vi "Read Component.vi"(6 "Create if non-existent? (F)":bool, 8 "error in (no error)":errorcluster, 10 "Qualified Path":string, 11 "Attribute.Identity in":refnum<class "Attribute.Identity.lvclass">) -> (0 "error out":errorcluster, 2 "Component":string, 3 "Attribute.Identity out":refnum<class "Attribute.Identity.lvclass">)   [LabVIEW 2013, in "Attribute.Identity.lvclass"]
uses:
  Attribute.Identity.lvclass
  Attribute.Identity.lvclass/Attribute.Identity.ctl
  <vilib>/Utility/MD5Checksum.llb/MD5Checksum string.vi
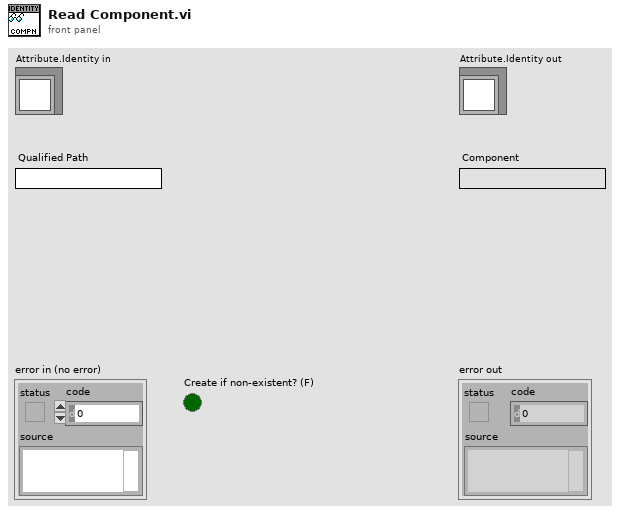
[diagram p1: front panel]
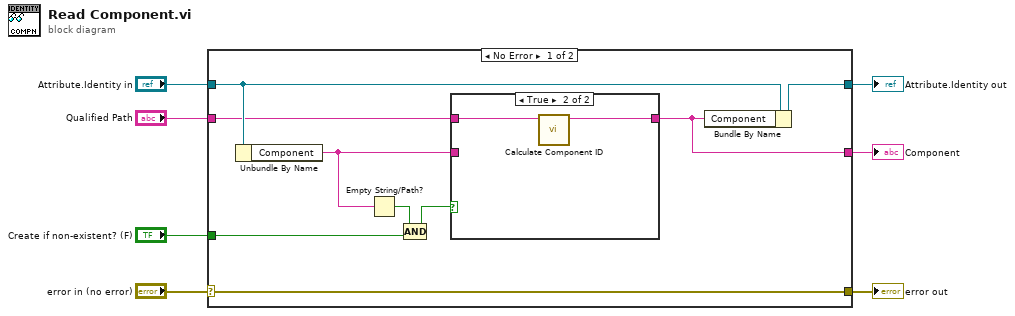
[diagram p0: block diagram]
diagram:
  n1 = case shown="No Error" "error in (no error)" {
    selector: "error in (no error)" -> [w16 w20]
    tunnel: [w16 w20] -> w6
    tunnel: [w9 w21] -> w4
    tunnel: "Attribute.Identity in" -> [w10 w21]
    tunnel: [w11 _] -> w3
    tunnel: "Create if non-existent? (F)" -> [w15 _]
    tunnel: "Qualified Path" -> [w8 _]
    frame No Error {
      n2 = Unbundle By Name(w10) -> ("Component"=w12:string)
      n3 = Empty String/Path?(string/path=w12) -> (empty?=w14:bool)
      n4 = Compound Arithmetic op=AND(w14, w15) -> (w13:bool)
      n5 = case shown="True" w13 {
        tunnel: w12 -> [w17 _]
        tunnel: [w17 w19] -> w11
        tunnel: w8 -> [_ w18]
        frame False {
        }
        frame True {
          n6 = call "Calculate Component ID.vi"("Input"=w18) -> ("Component ID"=w19:string)  [unwired: 10 in]
        }
      }
      n7 = Bundle By Name(cluster=w10, "Component"=w11) -> (w9:refnum<class "Attribute.Identity.lvclass">)
    }
    frame Error {
    }
  }
  "error out" <- w6
  "Attribute.Identity out" <- w4
  "Component" <- w3
